vi "Initialize Threads.vi"(5 "FIFO Options":T1, 7 "plugin configuration":T2={"name"="", "components"=[], "cycle timing"={"priority"=0, "decimation"=1, "offset"=0}, "threads"=[], "Transfer Groups"=[], "settings"=[]} {"Transfer Groups"."Transfers"."channels"."string offset" format="%d bytes"}, 8 "error in (no error)":errorcluster, 9 "component objects":refnum<class>[](array[class]), 10 "Transfer Groups":refnum<class "Transfer Group.lvclass">[](array[class]), 11 "Plugin in":refnum<class "Plugin.lvclass">) -> (0 "error out":errorcluster, 2 "Plugin Threads":refnum<class "Plugin Thread.lvclass">[](array[class]), 3 "Plugin out":refnum<class "Plugin.lvclass">)   [LabVIEW 2017, in "DSF Core.lvlib" / "Plugin.lvclass"]
uses:
  Plugin.lvclass
  Typedefs/DSF Engine Plugin Configuration.ctl
  Typedefs/DSF Timing Info.ctl
  Typedefs/DSF Engine Plugin Thread Configuration.ctl
  Typedefs/DSF Settings Info.ctl
  Typedefs/DSF Engine Transfer Group Configuration.ctl
  Typedefs/DSF Direction.ctl
  Typedefs/DSF Engine Transfer Configuration.ctl
  Typedefs/DSF Byte Order.ctl
  Typedefs/DSF Engine Channel Configuration.ctl
  Typedefs/DSF Data Type.ctl
  Typedefs/DSF Timeout Behavior.ctl
  Typedefs/DSF FIFO Options.ctl
  Thread/Plugin/Plugin Thread.lvclass
  C:/Git/DSF/Data Sharing Framework/Source/Core/Engine/Classes/Thread/Thread.lvclass
  Transfer Group/Transfer Group.lvclass
  Plugin.lvclass/Plugin.ctl
  Timing/Timing.lvclass/Timing.ctl
  Thread/Thread Settings.ctl
  Thread/Thread.lvclass/Thread.ctl
  Buffer Converter/Buffer Converter.lvclass
  Transceiver/Transceiver.lvclass
  Timing/Timing.lvclass
  Thread/Thread.lvclass
  Thread Pool/Plugin Interface Pool.lvclass
  DSF Core.lvlib
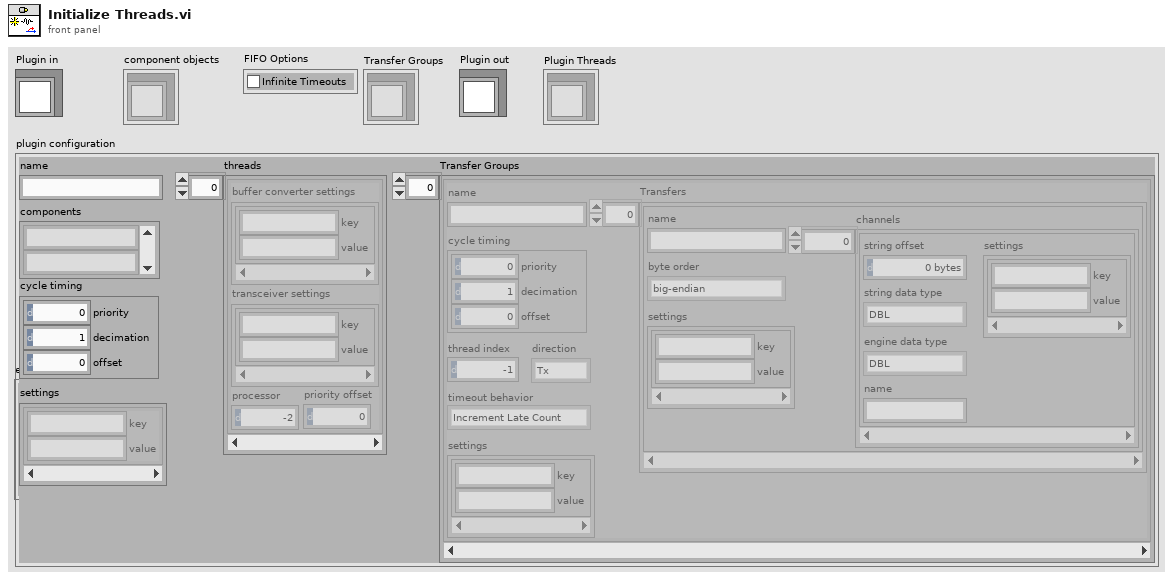
[diagram p1: front panel]
types:
  T1 = typedef "DSF Core.lvlib/DSF FIFO Options.ctl" = cluster{"Infinite Timeouts":bool}
  T2 = typedef "DSF Core.lvlib/DSF Engine Plugin Configuration.ctl" = cluster{"name":string, "components":string[], "cycle timing":T3, "threads":T4[], "Transfer Groups":T6[], "settings":T5}
  T3 = typedef "DSF Core.lvlib/DSF Timing Info.ctl" = cluster{"priority":u64, "decimation":u64, "offset":u64}
  T4 = typedef "DSF Core.lvlib/DSF Engine Plugin Thread Configuration.ctl" = cluster{"buffer converter settings":T5, "transceiver settings":T5, "processor":i32, "priority offset":i16}
  T5 = typedef "DSF Core.lvlib/DSF Settings Info.ctl" = cluster{"key":string, "value":string}[]
  T6 = typedef "DSF Core.lvlib/DSF Engine Transfer Group Configuration.ctl" = cluster{"name":string, "direction":T7, "cycle timing":T3, "thread index":i32, "settings":T5, "Transfers":T8[], "timeout behavior":T12}
  T7 = typedef "DSF Core.lvlib/DSF Direction.ctl" = enum8{"Tx", "Rx"}
  T8 = typedef "DSF Core.lvlib/DSF Engine Transfer Configuration.ctl" = cluster{"name":string, "byte order":T9, "settings":T5, "channels":T10[]}
  T9 = typedef "DSF Core.lvlib/DSF Byte Order.ctl" = enum8{"big-endian", "little-endian"}
  T10 = typedef "DSF Core.lvlib/DSF Engine Channel Configuration.ctl" = cluster{"string offset":u64, "string data type":T11, "engine data type":T11, "name":string, "settings":T5}
  T11 = typedef "DSF Core.lvlib/DSF Data Type.ctl" = enum8{"Bool", "SGL", "DBL", "I8", "I16", "I32", "I64", "U8", "U16", "U32", "U64"}
  T12 = typedef "DSF Core.lvlib/DSF Timeout Behavior.ctl" = enum8{"Increment Late Count", "Throw Error"}
  T13 = typedef "DSF Core.lvlib/Thread.lvclass/Thread Settings.ctl" = cluster{"Priority":u16, "Processor":i32, "ID":i32}
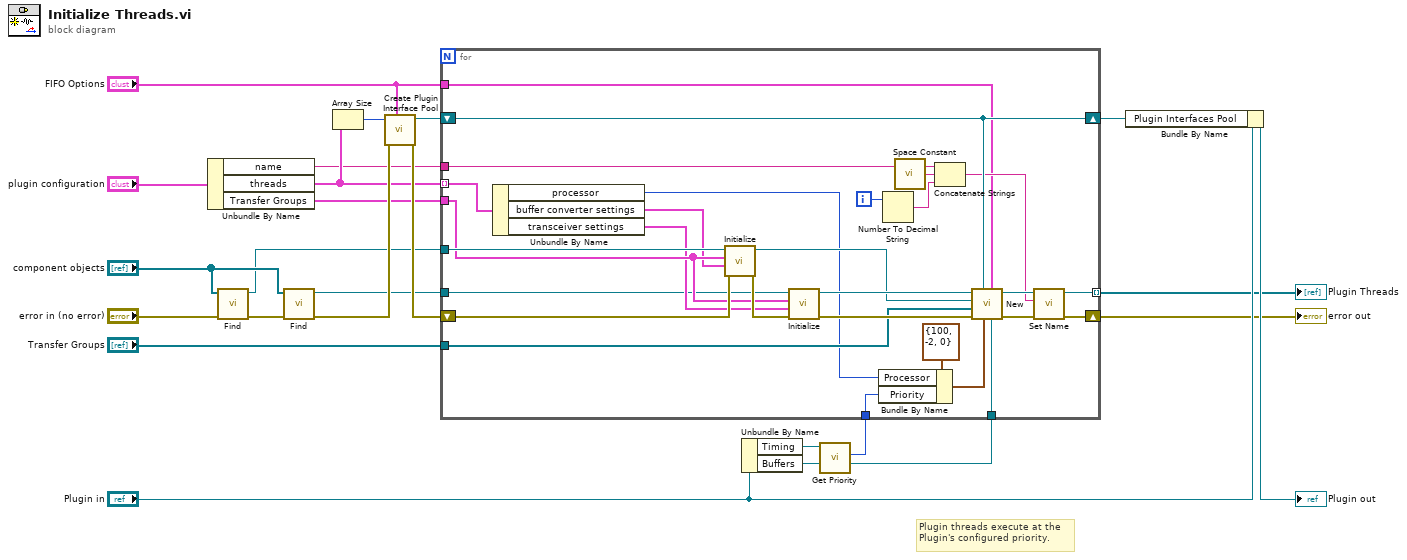
[diagram p0: block diagram]
diagram:
  # "Plugin threads execute at the Plugin's configured priority."
  n1 = Unbundle By Name("plugin configuration") -> ("name"=w1:string, "threads"=w4:T4[], "Transfer Groups"=w2:T6[])
  n2 = call "Find.vi"("error in (no error)"="error in (no error)", "component objects"="component objects") -> ("error out"=w21:errorcluster, "Buffer Converter"=w3:refnum<class "Buffer Converter.lvclass">)  [unwired: 7 in, 1 out]
  n3 = call "Find.vi"("error in (no error)"=w21, "component objects"="component objects") -> ("error out"=w23:errorcluster, "Transceiver"=w5:refnum<class "Transceiver.lvclass">)  [unwired: 7 in, 1 out]
  n4 = Array Size(array=w4) -> (size(s)=w6:i32)
  n5 = call "Create Plugin Interface Pool.vi"("FIFO Options"="FIFO Options", "error in (no error)"=w23, "number of interfaces"=w6) -> ("error out"=w22:errorcluster, "Plugin Thread Pool out"=w13:refnum<class "Plugin Interface Pool.lvclass">)  [unwired: 7 in]
  n6 = Unbundle By Name("Plugin in") -> ("Timing"=w18:refnum<class "Timing.lvclass">, "Buffers"=w12:refnum<class "Buffers.lvclass">)
  n7 = call "Get Priority.vi"("Timing in"=w18) -> ("Priority"=w17:u16)  [unwired: 9 in, 1 out]
  n8 = for {
    shift-right: [w50] -> w10
    shift-left: w22 -> [w35]
    tunnel: "Transfer Groups" -> [w29]
    tunnel: [w45] -> w14 mode=indexing
    tunnel: "FIFO Options" -> [w41]
    tunnel: w1 -> [w25]
    tunnel: w17 -> [w39]
    shift-right: [w49] -> w11
    shift-left: w13 -> [w49]
    tunnel: w12 -> [w42]
    tunnel: w4 -> [w37] mode=indexing
    tunnel: w3 -> [w36]
    tunnel: w5 -> [w26]
    tunnel: w2 -> [w32]
    i -> [w48]
    n9 = Unbundle By Name(w37) -> ("processor"=w24:i32, "buffer converter settings"=w27:T5, "transceiver settings"=w28:T5)
    n10 = call-dynamic "Initialize.vi"("error in (no error)"=w35, "settings"=w27, "Transfer Groups Configurations"=w32, "Buffer Converter in"=w36) -> ("error out"=w34:errorcluster, "Buffer Converter out"=w30:refnum<class "Buffer Converter.lvclass">)  [unwired: 6 in]
    n11 = call-dynamic "Initialize.vi"("error in (no error)"=w34, "settings"=w28, "Transfer Groups Configurations"=w32, "Transceiver in"=w26) -> ("error out"=w33:errorcluster, "Transceiver out"=w31:refnum<class "Transceiver.lvclass">)  [unwired: 6 in]
    n12 = Bundle By Name(cluster=T13 {"Priority"=100, "Processor"=-2, "ID"=0} ("thread settings"), "Processor"=w24, "Priority"=w39) -> (w38:T13)
    n13 = Number To Decimal String(number=w48) -> (decimal integer string=w47:string)  [unwired: 1 in]
    n14 = call <vilib>:"Space Constant.vi"() -> ("String"=w44:string)
    n15 = Concatenate Strings(w25, w44, w47) -> (w43:string)
    n16 = call "New.vi"("Buffers"=w42, "FIFO Options"=w41, "thread settings"=w38, "Plugin Interfaces Pool"=w49, "error in (no error)"=w33, "Transfer Groups"=w29, "Buffer Converter"=w30, "Transceiver"=w31) -> ("error out"=w50:errorcluster, "Plugin Thread out"=w46:refnum<class "Plugin Thread.lvclass">)  [unwired: 1 in, 1 out]
    n17 = call "Set Name.vi"("name"=w43, "Thread in"=w46) -> ("Thread out"=w45:refnum<class "Plugin Thread.lvclass">)  [unwired: 9 in]
  }
  "error out" <- w10
  "Plugin Threads" <- w14
  n18 = Bundle By Name(cluster="Plugin in", "Plugin Interfaces Pool"=w11) -> (→"Plugin out":refnum<class "Plugin.lvclass">)
